vi "Set_sourceItems.vi"(8 "error in (no error)":errorcluster, 10 "sourceItems":refnum<class "AB_Source.lvclass">[](array[class]), 11 "Class in":refnum<class "AB_Build.lvclass">) -> (0 "error out":errorcluster, 3 "Class out":refnum<class "AB_Build.lvclass">)   [LabVIEW 2020, in "AB_Build.lvclass"]
uses:
  <vilib>/AppBuilder/AB_Classes/Build/AB_Build.lvclass
  <vilib>/AppBuilder/AB_Classes/Source/AB_Source.lvclass
  <vilib>/AppBuilder/AB_Classes/Build/AB_Build.lvclass/AB_Build.ctl
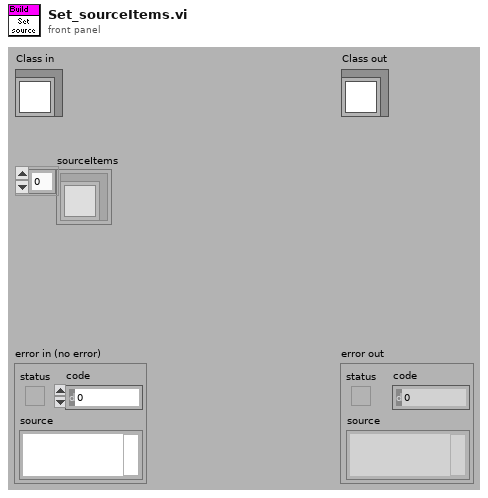
[diagram p1: front panel]
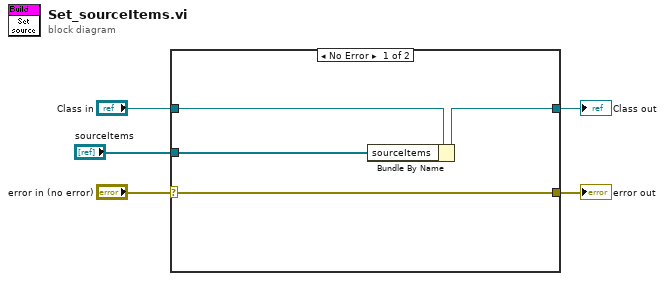
[diagram p0: block diagram]
diagram:
  n1 = case "Case" shown="No Error" "error in (no error)" {
    selector: "error in (no error)" -> [w9 w11]
    tunnel: [w9 w11] -> w4
    tunnel: [w8 w10] -> w2
    tunnel: "Class in" -> [w7 w10]
    tunnel: "sourceItems" -> [w6 _]
    frame No Error {
      n2 = Bundle By Name(cluster=w7, "sourceItems"=w6) -> (w8:refnum<class "AB_Build.lvclass">)
    }
    frame Error {
    }
  }
  "error out" <- w4
  "Class out" <- w2
